vi "test controllers.vi"() -> ()   [LabVIEW 2016]
uses:
  Classes/Controller/Motion/A3200 Folder/A3200.lvclass
  D:/Gantry_General/Classes/Controller/Motion/Motion Folder/Motion.lvclass
  Classes/Controller/Dispenser/Ultimus V2 Folder/Ultimus V2.lvclass
  Classes/Controller/I-O/NI-DAQ Folder/NI-DAQ.lvclass
  D:/Gantry_General/Classes/Controller/I-O/I-O Folder/I-O.lvclass
  Classes/Controller/Motion/Motion Folder/Motion.lvclass
  Classes/Controller/I-O/I-O Folder/I-O.lvclass
  Classes/Controller/Dispenser/Dispenser Folder/Dispenser.lvclass
panel:
  in  "n":i32
  out "Array":u32[][](array[numeric])
  in  "milliseconds to wait":u32
  in  "delay time test":bool
  out "Array 2":bool[](array[boolean])
  out "XYZTheta Out":dbl[](array[numeric]) format="%#_8g"
  out "Numeric":dbl
  in  "Tab Control":T1(tab)=enum."IO"
  in  "U angle":dbl format="%#_13g"
  in  "XYZU":dbl[](array[numeric])=[898.0, 787.0, 0.0, 0.0]
  in  "XYZU Go":bool
  in  "Abs XY Go":bool
  in  "XY":dbl[](array[numeric])=[100.0, 100.0]
  in  "Lower  test":bool
  in  "Z Speed":dbl=5.0 format="%#_13g"
  in  "Position":dbl format="%#_13g"
  in  "Z Go":bool
  in  "Lower stop":bool
  in  "Lower stop ms":bool
  out "L run":bool
  out "L run ms":bool
  in  "Lower stop ms2":bool
  out "L run ms2":bool
  out "L run ms3t":bool
  in  "test joystick":bool
  in  "joystick":bool
  in  "joystick ms":bool
  in  "get xy center":bool
  out "XY theta out":dbl
  out "offset P1-P2":dbl[](array[numeric])
  out "XY center out":dbl[](array[numeric])=[898.8680246146163, 787.774390745643]
  in  "dispenser change":bool
  in  "Pressure":i16
  in  "Vacuum Setting (0000)":i64 min=0 max=1000 step=1 format="%04.0f"
  in  "IO control":bool
  in  "indices":i32[](array[numeric])
  in  "values":bool[](array[boolean])
  in  "IO turn off":bool
  in  "controller":T2
  in  "stop":bool
  # "bug： \nchange value fail \nevent delay"
  # "bug： \n持續移動距離過多"
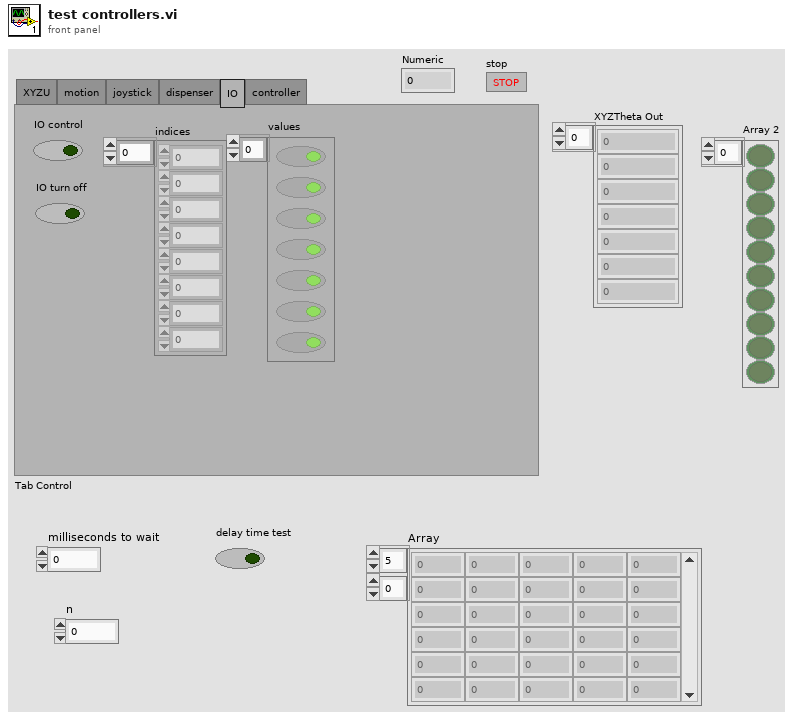
[diagram p1: front panel]
types:
  T1 = enum32{"XYZU", "motion", "joystick", "dispenser", "IO", "controller"}
  T2 = cluster{"A3200.lvclass":refnum<class "A3200.lvclass">, "Ultimus V2.lvclass":refnum<class "Ultimus V2.lvclass">, "NI-DAQ.lvclass":refnum<class "NI-DAQ.lvclass">, "Motion.lvclass":refnum<class "Motion.lvclass">, "I-O.lvclass":refnum<class "I-O.lvclass">, "Dispenser.lvclass":refnum<class "Dispenser.lvclass">}
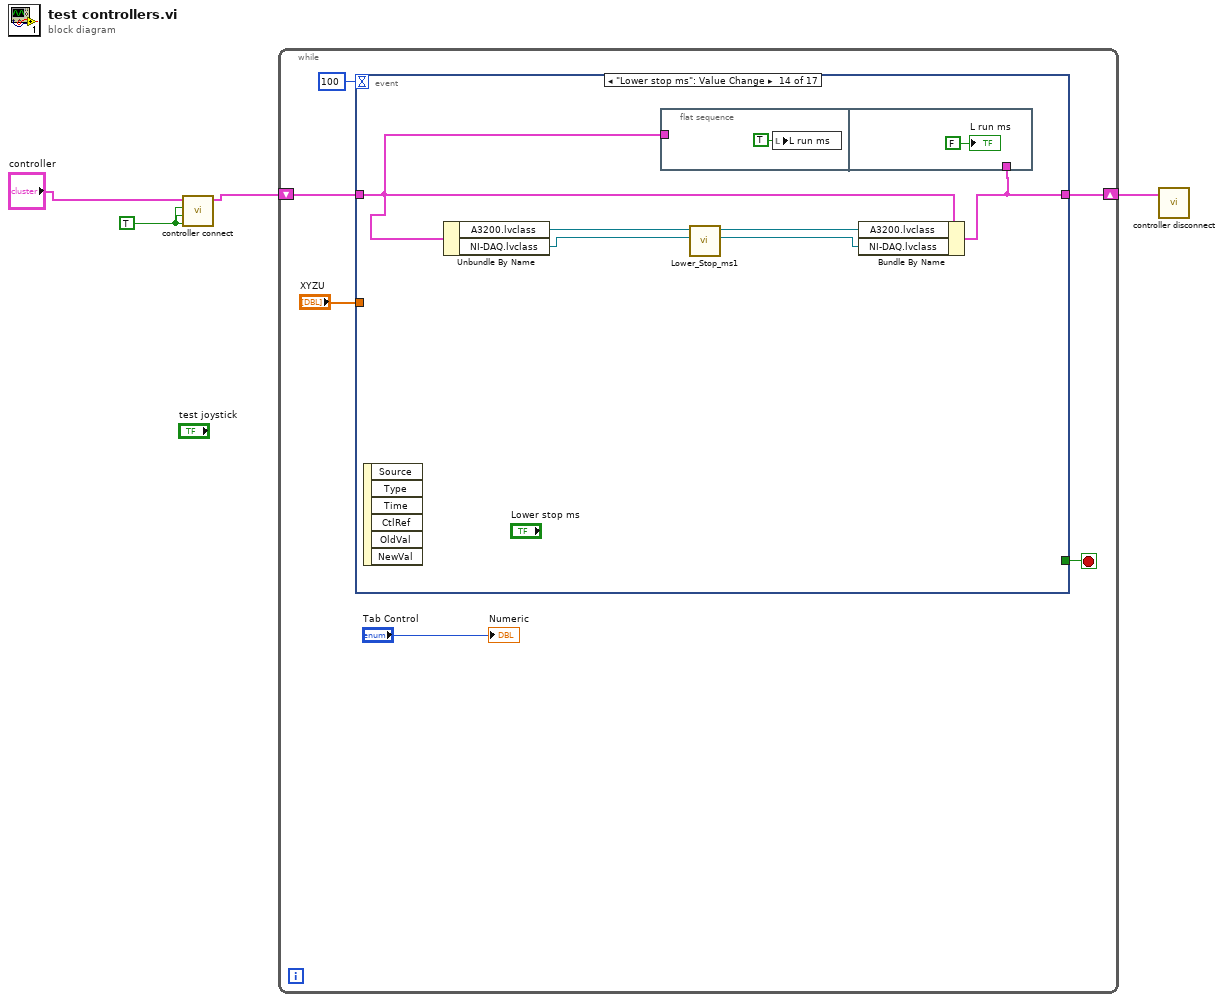
[diagram p0: block diagram]
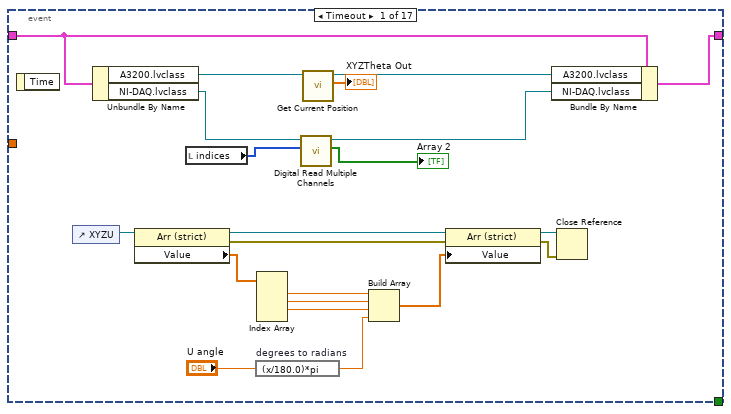
[diagram p2: hidden frame]
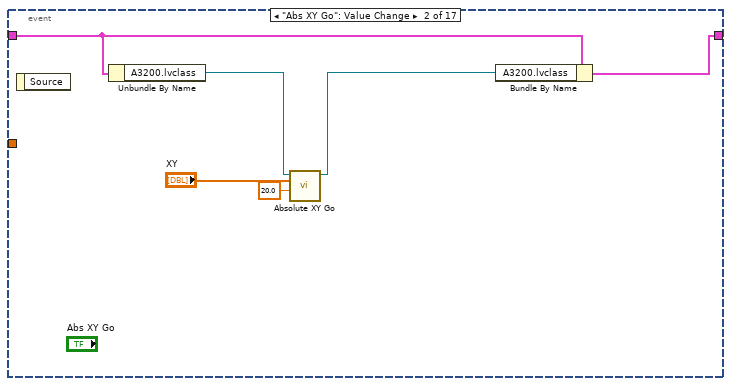
[diagram p3: hidden frame]
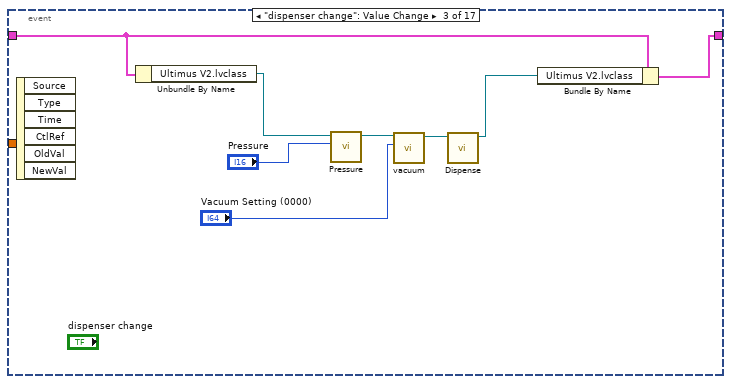
[diagram p4: hidden frame]
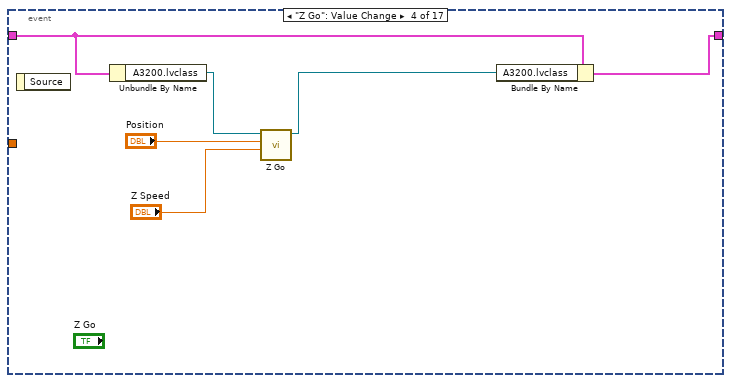
[diagram p5: hidden frame]
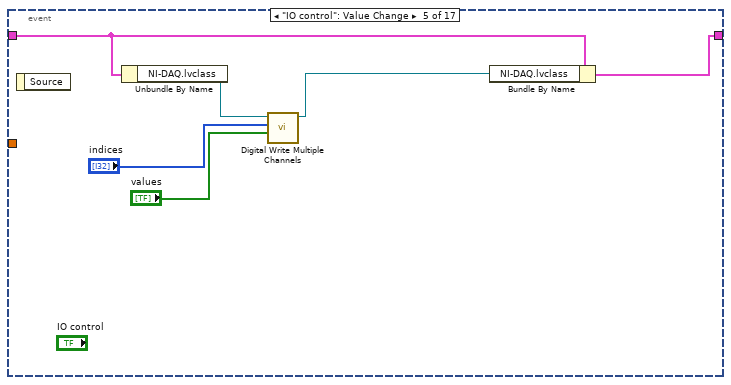
[diagram p6: hidden frame]
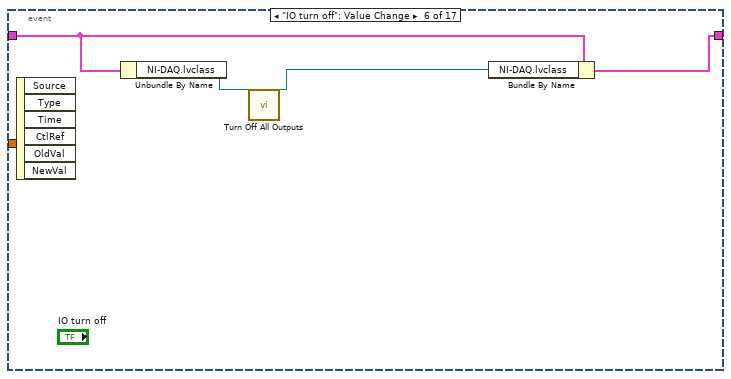
[diagram p7: hidden frame]
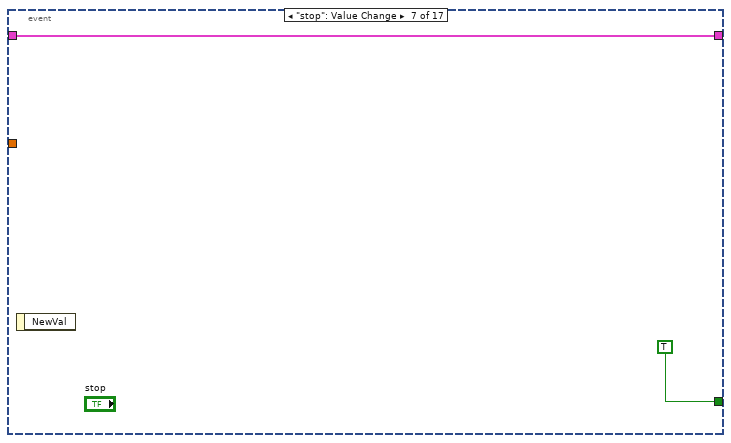
[diagram p8: hidden frame]
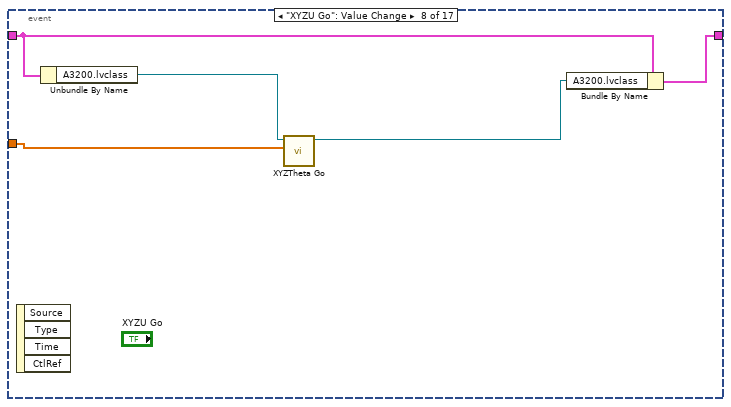
[diagram p9: hidden frame]
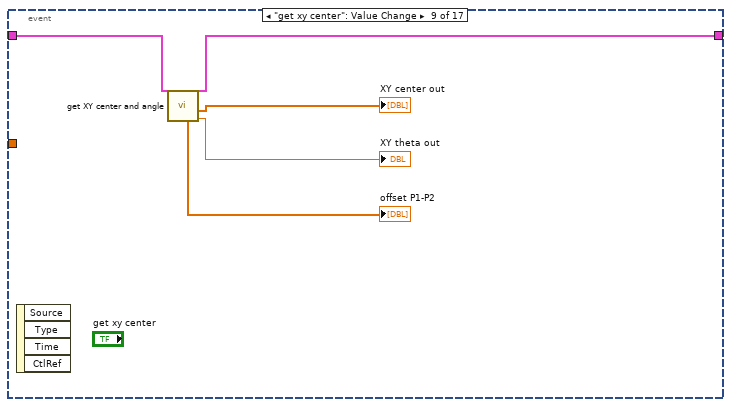
[diagram p10: hidden frame]
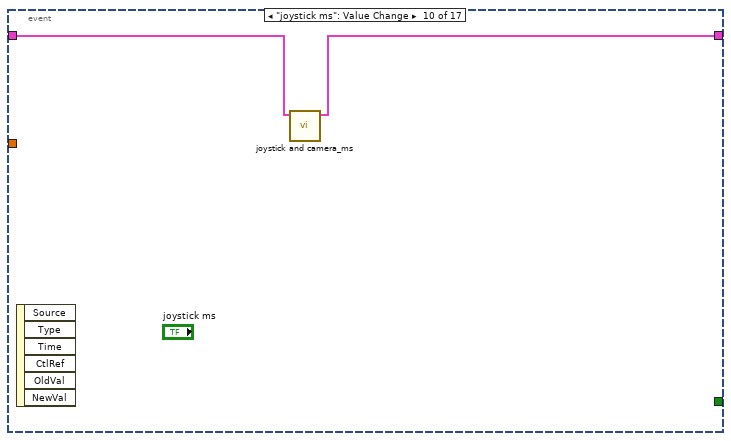
[diagram p11: hidden frame]
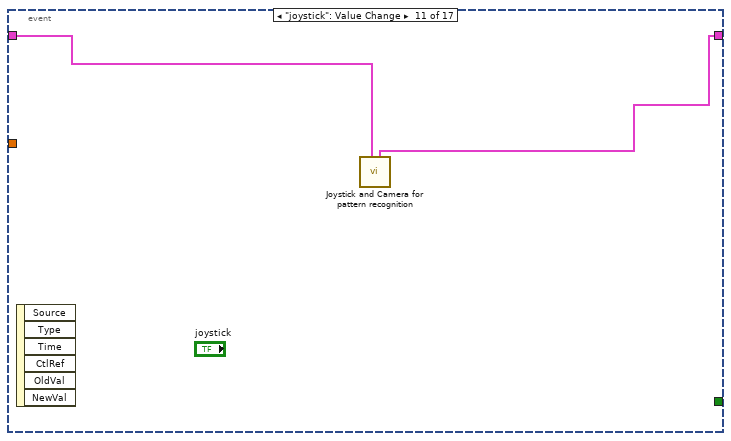
[diagram p12: hidden frame]
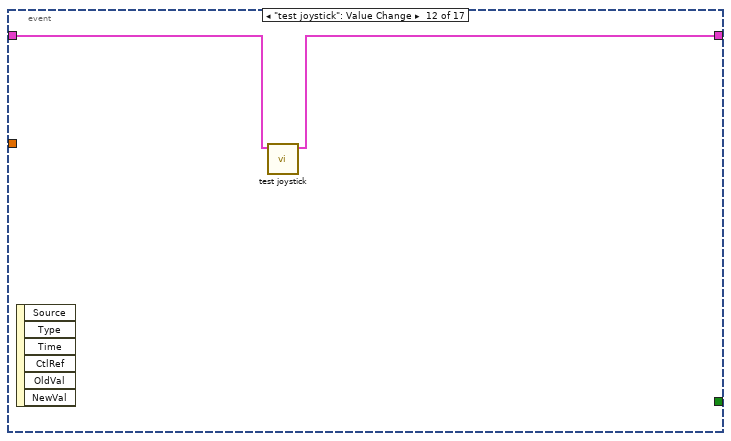
[diagram p13: hidden frame]
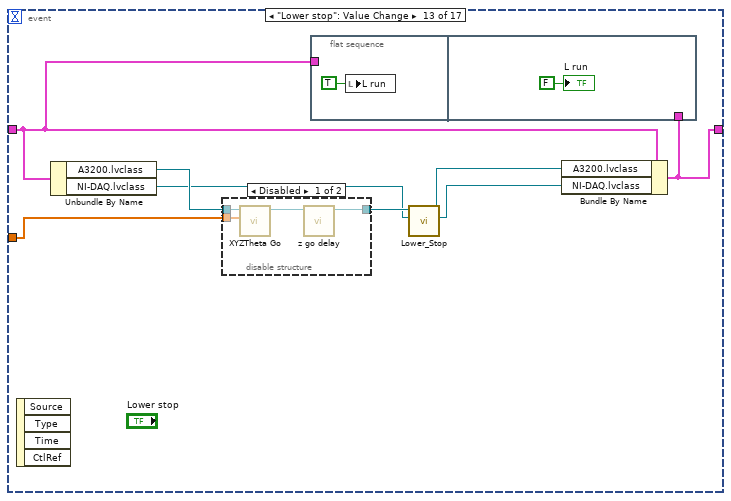
[diagram p14: hidden frame]
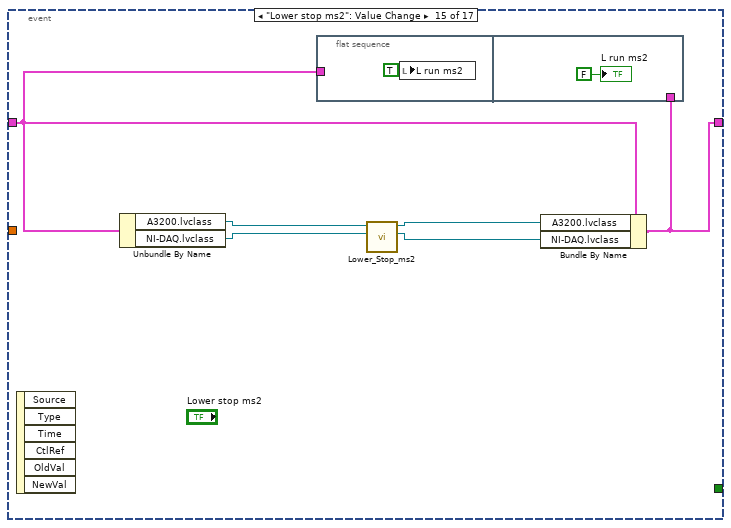
[diagram p16: hidden frame]
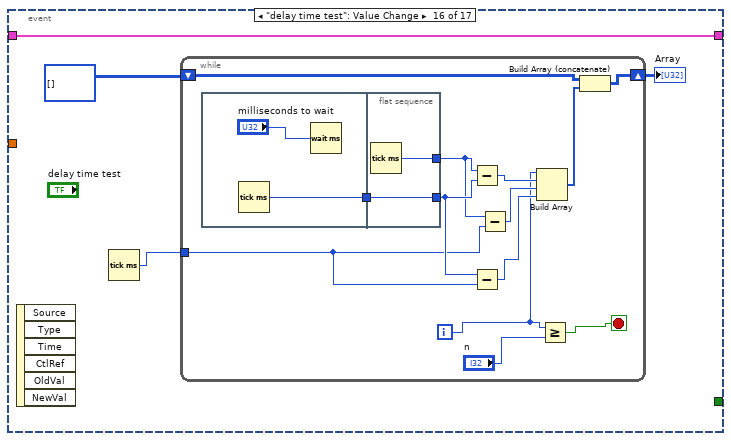
[diagram p17: hidden frame]
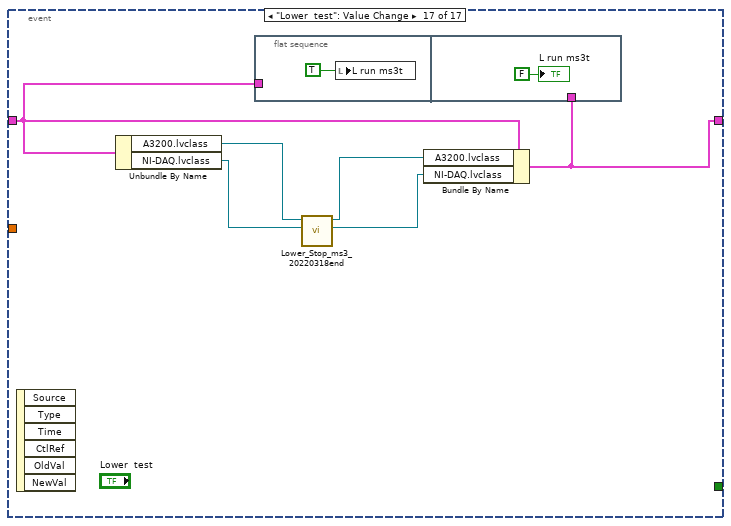
[diagram p18: hidden frame]
diagram:
  w4 = TRUE ("IO on")
  n1 = call "controller connect.vi"("IO on"=w4, "dispencer on"=w4, "motion on"=w4, "controller in"="controller") -> ("controller out"=w3:T2)  [unwired: 7 in]
  n2 = while {
    shift-right: [w7] -> w2
    shift-left: w3 -> [w8]
    stop <- w10 stop-if-true
    n3 = event shown="[13] \"Lower stop ms\": Value Change" {
      selector: _ -> [_ _ _ _ _ _ _ _ _ _ _ _ _ _ _ _ _]
      dyn-events: _ -> [_ _ _ _ _ _ _ _ _ _ _ _ _ _ _ _ _]
      timeout: 100 -> [_ _ _ _ _ _ _ _ _ _ _ _ _ _ _ _ _]
      tunnel: [_ _ _ _ _ _ TRUE _ _ _ _ _ _ _ _ _ _] -> w10
      tunnel: w8 -> [w31 w33 w45 w49 w57 w61 w62 w68 w73 w75 w77 w79 w81 w96 w105 w114 w136]
      tunnel: [w30 w32 w44 w48 w56 w60 w62 w67 w72 w74 w76 w78 w80 w95 w106 w114 w137] -> w7
      tunnel: "XYZU" -> [_ _ _ _ _ _ _ w64 _ _ _ _ w82 _ _ _ _]
      event Timeout {
        n4 = event-data() -> ()  [unwired: 1 in, 1 out]
        n5 = control-ref of="XYZU"() -> (w14:refnum<vi>)
        n6 = Unbundle By Name(w31) -> ("A3200.lvclass"=w25:refnum<class "A3200.lvclass">, "NI-DAQ.lvclass"=w27:refnum<class "NI-DAQ.lvclass">)
        n7 = property class="Arr (strict)"(reference=w14) -> (reference out=w13:refnum<vi>, error out=w12:errorcluster, "Value"=w11:dbl[])  [unwired: 1 in]
        n8 = local read "indices"() -> (w26:i32[])
        n9 = expression code="(x/180.0)*pi" "degrees to radians"("U angle") -> (w17:dbl)
        n10 = Index Array(array=w11) -> (element #1=w21:dbl, element #2=w20:dbl, element #3=w19:dbl)  [unwired: 4 in, 1 out]
        n11 = call-dynamic "Digital Read Multiple Channels.vi"("Array"=w26, "NI-DAQ in"=w27) -> ("subarray"=→"Array 2":bool[], "NI-DAQ out"=w28:refnum<class "NI-DAQ.lvclass">)  [unwired: 7 in, 1 out]
        n12 = call-dynamic "Get Current Position.vi"("Gantry in"=w25) -> ("XYZTheta Out"=→"XYZTheta Out":dbl[], "Gantry out"=w24:refnum<class "A3200.lvclass">)  [unwired: 8 in, 1 out]
        n13 = Build Array(w21, w20, w19, w17) -> (w22:dbl[])
        n14 = property class="Arr (strict)"(reference=w13, error in=w12, "Value"=w22) -> (reference out=w15:refnum<vi>, error out=w16:errorcluster)
        n15 = Bundle By Name(cluster=w31, "A3200.lvclass"=w24, "NI-DAQ.lvclass"=w28) -> (w30:T2)
        n16 = Close Reference(reference=w15, error in (no error)=w16) -> ()  [unwired: 1 out]
      }
      event "Abs XY Go": Value Change {
        n17 = event-data() -> ()  [unwired: 1 in, 1 out]
        n18 = Unbundle By Name(w33) -> ("A3200.lvclass"=w35:refnum<class "A3200.lvclass">)
        n19 = call-dynamic "Absolute XY Go.vi"("Speed"=20.0, "XY"="XY", "Gantry in"=w35) -> ("Gantry out"=w34:refnum<class "A3200.lvclass">)  [unwired: 7 in, 1 out]
        n20 = Bundle By Name(cluster=w33, "A3200.lvclass"=w34) -> (w32:T2)
      }
      event "dispenser change": Value Change {
        n21 = event-data() -> ()  [unwired: 1 in, 6 out]
        n22 = Unbundle By Name(w45) -> ("Ultimus V2.lvclass"=w41:refnum<class "Ultimus V2.lvclass">)
        n23 = call-dynamic "Pressure.vi"("Pressure"="Pressure", "Ultimus V in"=w41) -> ("Ultimus V out"=w40:refnum<class "Ultimus V2.lvclass">)  [unwired: 8 in, 1 out]
        n24 = call "vacuum.vi"("Vacuum Setting (0000)"="Vacuum Setting (0000)", "Ultimus V in"=w40) -> ("Ultimus V out"=w39:refnum<class "Ultimus V2.lvclass">)  [unwired: 8 in, 1 out]
        n25 = call-dynamic "Dispense.vi"("Ultimus V in"=w39) -> ("Ultimus V out"=w38:refnum<class "Ultimus V2.lvclass">)  [unwired: 9 in, 1 out]
        n26 = Bundle By Name(cluster=w45, "Ultimus V2.lvclass"=w38) -> (w44:T2)
      }
      event "Z Go": Value Change {
        n27 = event-data() -> ()  [unwired: 1 in, 1 out]
        n28 = Unbundle By Name(w49) -> ("A3200.lvclass"=w50:refnum<class "A3200.lvclass">)
        n29 = call-dynamic "Z Go.vi"("Speed"="Z Speed", "Position"="Position", "Gantry in"=w50) -> ("Gantry out"=w47:refnum<class "A3200.lvclass">)  [unwired: 7 in, 1 out]
        n30 = Bundle By Name(cluster=w49, "A3200.lvclass"=w47) -> (w48:T2)
      }
      event "IO control": Value Change {
        n31 = event-data() -> ()  [unwired: 1 in, 1 out]
        n32 = Unbundle By Name(w57) -> ("NI-DAQ.lvclass"=w55:refnum<class "NI-DAQ.lvclass">)
        n33 = call-dynamic "Digital Write Multiple Channels.vi"("Values"="values", "Indices"="indices", "NI-DAQ in"=w55) -> ("NI-DAQ out"=w52:refnum<class "NI-DAQ.lvclass">)  [unwired: 7 in, 1 out]
        n34 = Bundle By Name(cluster=w57, "NI-DAQ.lvclass"=w52) -> (w56:T2)
      }
      event "IO turn off": Value Change {
        n35 = event-data() -> ()  [unwired: 1 in, 6 out]
        n36 = Unbundle By Name(w61) -> ("NI-DAQ.lvclass"=w59:refnum<class "NI-DAQ.lvclass">)
        n37 = call-dynamic "Turn Off All Outputs.vi"("NI-DAQ in"=w59) -> ("NI-DAQ out"=w58:refnum<class "NI-DAQ.lvclass">)  [unwired: 9 in, 1 out]
        n38 = Bundle By Name(cluster=w61, "NI-DAQ.lvclass"=w58) -> (w60:T2)
      }
      event "stop": Value Change {
        n39 = event-data() -> ()  [unwired: 1 in, 1 out]
      }
      event "XYZU Go": Value Change {
        n40 = event-data() -> ()  [unwired: 1 in, 4 out]
        n41 = Unbundle By Name(w68) -> ("A3200.lvclass"=w65:refnum<class "A3200.lvclass">)
        n42 = call "XYZTheta Go.vi"("XYZTheta In"=w64, "Motion in"=w65) -> ("Motion out"=w66:refnum<class "A3200.lvclass">)  [unwired: 7 in, 2 out]
        n43 = Bundle By Name(cluster=w68, "A3200.lvclass"=w66) -> (w67:T2)
      }
      event "get xy center": Value Change {
        n44 = event-data() -> ()  [unwired: 1 in, 4 out]
        n45 = call "get XY center and angle.vi"("controller in"=w73) -> ("XY theta out"=→"XY theta out":dbl, "XY center out"=→"XY center out":dbl[], "controller out"=w72:T2, "offset P1-P2"=→"offset P1-P2":dbl[])  [unwired: 7 in]
      }
      event "joystick ms": Value Change {
        n46 = event-data() -> ()  [unwired: 1 in, 6 out]
        n47 = call "joystick and camera_ms.vi"("controller in"=w75) -> ("controller out"=w74:T2)  [unwired: 9 in, 1 out]
      }
      event "joystick": Value Change {
        n48 = event-data() -> ()  [unwired: 1 in, 6 out]
        n49 = call "Joystick and Camera for pattern recognition.vi"("controller in"=w77) -> ("controller out"=w76:T2)  [unwired: 7 in, 3 out]
      }
      event "test joystick": Value Change {
        n50 = event-data() -> ()  [unwired: 1 in, 6 out]
        n51 = call "test joystick .vi"("controller IN"=w79) -> ("controller OUT"=w78:T2)  [unwired: 10 in]
      }
      event "Lower stop": Value Change {
        n52 = event-data() -> ()  [unwired: 1 in, 4 out]
        n53 = Unbundle By Name(w81) -> ("A3200.lvclass"=w87:refnum<class "A3200.lvclass">, "NI-DAQ.lvclass"=w85:refnum<class "NI-DAQ.lvclass">)
        n54 = disable-structure shown="Disabled" {
          disable-tunnel: w87 -> [w92 w94]
          disable-tunnel: [w91 w94] -> w86
          disable-tunnel: w82 -> [w90 _]
          frame Disabled {
            n55 = call "XYZTheta Go.vi"("XYZTheta In"=w90, "Motion in"=w92) -> ("Motion out"=w93:refnum<class "A3200.lvclass">)  [unwired: 7 in, 2 out]
            n56 = call "z go delay.vi"("Motion.lvclass"=w93) -> ("Motion.lvclass 2"=w91:refnum<class "A3200.lvclass">)  [unwired: 10 in]
          }
          frame Enabled {
          }
        }
        n57 = flat-sequence {
          tunnel: w81 -> [_]
          tunnel: w80 -> [_]
          frame #0 {
            n58 = local write "L run"(TRUE ("L run")) -> ()
          }
          frame #1 {
            "L run" <- FALSE ("L run")
          }
        }
        n59 = call "Lower_Stop.vi"("I-O in"=w85, "Motion in"=w86) -> ("I-O out"=w84:refnum<class "NI-DAQ.lvclass">, "Motion out"=w83:refnum<class "A3200.lvclass">)  [unwired: 7 in, 1 out]
        n60 = Bundle By Name(cluster=w81, "A3200.lvclass"=w83, "NI-DAQ.lvclass"=w84) -> (w80:T2)
      }
      event "Lower stop ms": Value Change {
        n61 = event-data() -> ()  [unwired: 1 in, 6 out]
        n62 = Unbundle By Name(w96) -> ("A3200.lvclass"=w100:refnum<class "A3200.lvclass">, "NI-DAQ.lvclass"=w99:refnum<class "NI-DAQ.lvclass">)
        n63 = flat-sequence {
          tunnel: w96 -> [_]
          tunnel: w95 -> [_]
          frame #0 {
            n64 = local write "L run ms"(TRUE ("L run 2")) -> ()
          }
          frame #1 {
            "L run ms" <- FALSE ("L run 2")
          }
        }
        n65 = call "Lower_Stop_ms1.vi"("I-O in"=w99, "Motion in"=w100) -> ("I-O out"=w98:refnum<class "NI-DAQ.lvclass">, "Motion out"=w97:refnum<class "A3200.lvclass">)  [unwired: 7 in, 1 out]
        n66 = Bundle By Name(cluster=w96, "A3200.lvclass"=w97, "NI-DAQ.lvclass"=w98) -> (w95:T2)
      }
      event "Lower stop ms2": Value Change {
        n67 = event-data() -> ()  [unwired: 1 in, 6 out]
        n68 = Unbundle By Name(w105) -> ("A3200.lvclass"=w108:refnum<class "A3200.lvclass">, "NI-DAQ.lvclass"=w107:refnum<class "NI-DAQ.lvclass">)
        n69 = flat-sequence {
          tunnel: w105 -> [_]
          tunnel: w106 -> [_]
          frame #0 {
            n70 = local write "L run ms2"(TRUE ("L run 3")) -> ()
          }
          frame #1 {
            "L run ms2" <- FALSE ("L run 3")
          }
        }
        n71 = call "Lower_Stop_ms2.vi"("I-O in"=w107, "Motion in"=w108) -> ("I-O out"=w104:refnum<class "NI-DAQ.lvclass">, "Motion out"=w103:refnum<class "A3200.lvclass">)  [unwired: 7 in, 1 out]
        n72 = Bundle By Name(cluster=w105, "A3200.lvclass"=w103, "NI-DAQ.lvclass"=w104) -> (w106:T2)
      }
      event "delay time test": Value Change {
        n73 = event-data() -> ()  [unwired: 1 in, 6 out]
        n74 = Tick Count (ms)() -> (millisecond timer value=w113:u32)
        n75 = while {
          tunnel: w113 -> [w124]
          shift-right: [w119] -> w112
          shift-left: u32[][] [] -> [w118]
          i -> [w116]
          stop <- w117 stop-if-true
          n76 = flat-sequence {
            tunnel: [w128] -> w126
            tunnel: [w131] -> w125
            tunnel: w126 -> [w131]
            tunnel: [w130] -> w123
            frame #0 {
              n77 = Tick Count (ms)() -> (millisecond timer value=w128:u32)
              n78 = Wait (ms)(milliseconds to wait="milliseconds to wait") -> ()  [unwired: 1 out]
            }
            frame #1 {
              n79 = Tick Count (ms)() -> (millisecond timer value=w130:u32)
            }
          }
          n80 = Subtract(x=w123, y=w125) -> (x-y=w127:u32)
          n81 = Subtract(x=w125, y=w124) -> (x-y=w121:u32)
          n82 = Subtract(x=w123, y=w124) -> (x-y=w122:u32)
          n83 = Build Array(w116, w127, w122, w121) -> (w120:u32[])
          n84 = Greater Or Equal?(x=w116, y="n") -> (x >= y?=w117:bool)
          n85 = Build Array (concatenate)(w118, w120) -> (w119:u32[][])
        }
        "Array" <- w112
      }
      event "Lower  test": Value Change {
        n86 = event-data() -> ()  [unwired: 1 in, 6 out]
        n87 = Unbundle By Name(w136) -> ("A3200.lvclass"=w135:refnum<class "A3200.lvclass">, "NI-DAQ.lvclass"=w132:refnum<class "NI-DAQ.lvclass">)
        n88 = flat-sequence {
          tunnel: w136 -> [_]
          tunnel: w137 -> [_]
          frame #0 {
            n89 = local write "L run ms3t"(TRUE ("L run 3")) -> ()
          }
          frame #1 {
            "L run ms3t" <- FALSE ("L run 3")
          }
        }
        n90 = call "Lower_Stop_ms3_20220318end.vi"("I-O in"=w132, "Motion in"=w135) -> ("I-O out"=w134:refnum<class "NI-DAQ.lvclass">, "Motion out"=w133:refnum<class "A3200.lvclass">)  [unwired: 7 in, 1 out]
        n91 = Bundle By Name(cluster=w136, "A3200.lvclass"=w133, "NI-DAQ.lvclass"=w134) -> (w137:T2)
      }
    }
    "Numeric" <- "Tab Control"
  }
  n92 = call "controller disconnect.vi"("controller 2"=w2) -> ()  [unwired: 11 in]
